vi "FM INIT.vi"   [LabVIEW 2009]
uses:
  MWC Global.vi
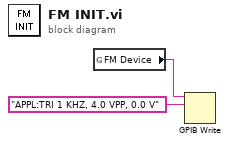
[diagram p0: block diagram]
diagram:
  n1 = global read "MWC Global.vi" "FM Device"() -> (w2:string)
  n2 = GPIB Write(0:w2, 1:"APPL:TRI 1 KHZ, 4.0 VPP, 0.0 V" ("data")) -> ()  [unwired: 3 in, 2 out]
